vi "CircularRadius.vi"(5 "Direction":u16(ring) items=["Clockwise", "Counter-clockwise"], 6 "radius":dbl format="%#_13g", 8 "error in (no error)":errorcluster, 9 "Speed":dbl format="%#_13g", 10 "XY End":dbl[](array[numeric]) format="%#_13g", 11 "A3200 in":refnum<class "A3200.lvclass">) -> (0 "error out":errorcluster, 3 "A3200 out":refnum<class "A3200.lvclass">)   [LabVIEW 2016, in "A3200.lvclass"]
uses:
  A3200.lvclass
  A3200.lvclass/A3200.ctl
  <userlib>/Aerotech A3200.lnk/Aerotech VIs.lvlib
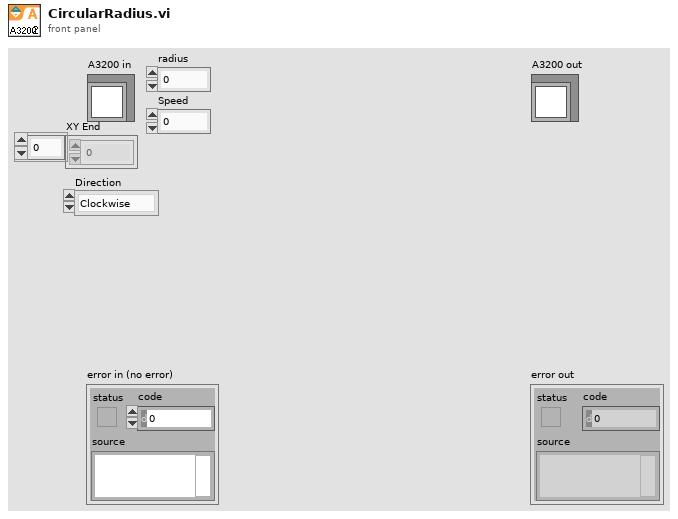
[diagram p1: front panel]
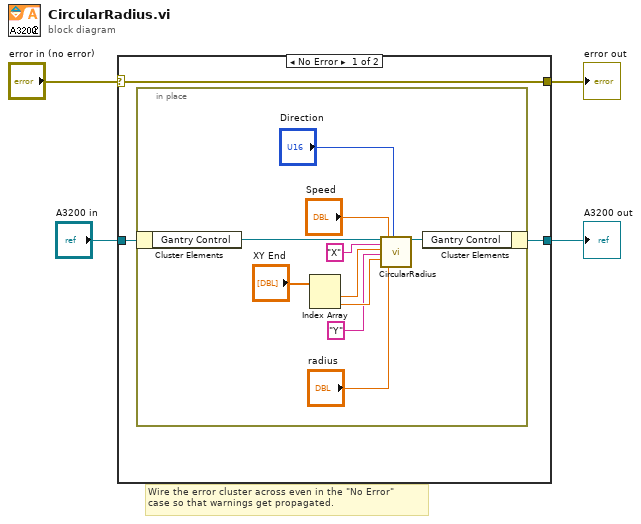
[diagram p0: block diagram]
diagram:
  # "Wire the error cluster across even in the \"No Error\"\ncase so that warnings get propagated."
  n1 = case shown="No Error" "error in (no error)" {
    selector: "error in (no error)" -> [w7 w19]
    tunnel: [w7 w19] -> w3
    tunnel: [w5 w18] -> w2
    tunnel: "A3200 in" -> [w6 w18]
    frame No Error {
      n2 = in-place {
        n3 = in-place-cluster #1(w6) -> ("Gantry Control"=w13:refnum<k24>)
        n4 = Index Array(array="XY End") -> (element #1=w16:dbl, element #2=w15:dbl)  [unwired: 2 in]
        n5 = call <userlib>:"CircularRadius.vi"("controller in"=w13, "axis 1 name"="X", "axis 1 endpoint"=w16, "axis 2 name"="Y" ("axis 1 name"), "axis 2 endpoint"=w15, "speed"="Speed", "radius"="radius", "direction"="Direction") -> ("controller out"=w12:refnum<k24>)  [unwired: 10 in, 1 out]
        n6 = in-place-cluster #1("Gantry Control"=w12) -> (w5:refnum<class "A3200.lvclass">)
      }
    }
    frame Error {
    }
  }
  "error out" <- w3
  "A3200 out" <- w2
